vi "Core Actor (ROOT) - Dispatch Message to Child (Nested_Actor).vi"(8 "error in (no error)":errorcluster, 11 "Child_6_Class in":refnum<class "Embedded_DB_Class.lvclass">) -> (0 "error out":errorcluster, 3 "Child_6_Class out":refnum<class "Embedded_DB_Class.lvclass">)   [LabVIEW 2023, in "Embedded_DB_Actor.lvlib" / "Embedded_DB_Class.lvclass"]
uses:
  Embedded_DB_Class.lvclass
  Abstraction_Interface_Class/Abstraction_Interface_Class.lvclass
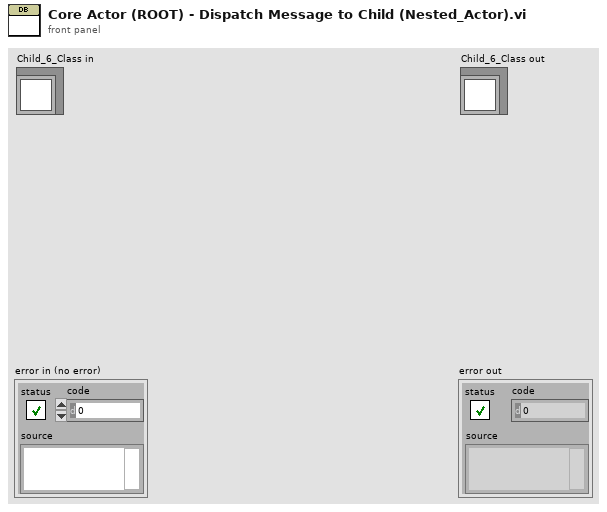
[diagram p1: front panel]
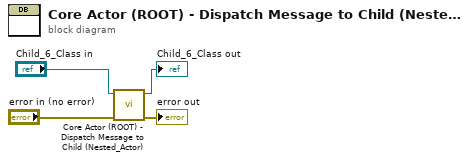
[diagram p0: block diagram]
diagram:
  n1 = call-parent "Core Actor (ROOT) - Dispatch Message to Child (Nested_Actor).vi"("error in (no error)"="error in (no error)", "Interface_Class in"="Child_6_Class in") -> ("error out"=→"error out":errorcluster, "Interface_Class out"=→"Child_6_Class out":refnum<class "Embedded_DB_Class.lvclass">)  [unwired: 8 in]
